vi "Wait n mSec.vi"(2 "Do Not Wait on Error?":bool=TRUE caption="Do NOT Wait on Error?\n(true)", 9 "Error in (no error)":errorcluster, 13 "Milliseconds to Wait (1)":u32=1 caption="mS") -> (10 "Error Out":errorcluster)   [LabVIEW 2015]
doc: "This VI allows you to drop in wait ms delays in your data-flow. Additionally it lets you specify if the wait should be skipped on errors (default) or if you want the wait to occur regardless of the error state!\nThe default wait value should be changed to suit your application."
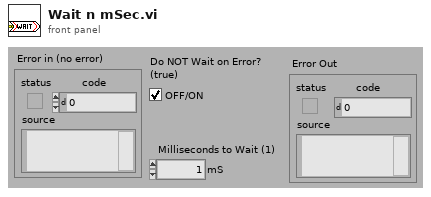
[diagram p1: front panel]
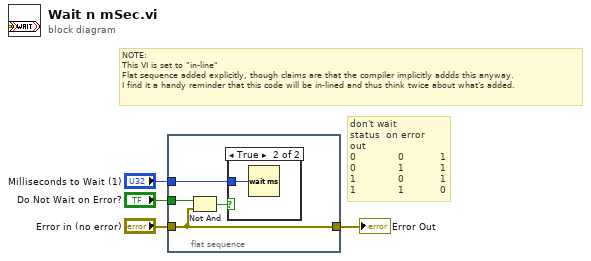
[diagram p0: block diagram]
diagram:
  # "don't wait  \nstatus  on error   out\n0              0            1\n0              1            1\n1              0            1\n1              1            0"
  # "NOTE:\nThis VI is set to \"in-line\"\nFlat sequence added explicitly, though claims are that the compiler implicitly addds this anyway.\nI find it a handy reminder that this code will be in-lined and thus think twice about what's added."
  n1 = flat-sequence {
    tunnel: "Milliseconds to Wait (1)" -> [w8]
    tunnel: [w6] -> w3
    tunnel: "Error in (no error)" -> [w6]
    tunnel: "Do Not Wait on Error?" -> [w7]
    frame #0 {
      n2 = Not And(1:w6, 2:w7) -> (0:w5:bool)
      n3 = case shown="True" w5 {
        tunnel: w8 -> [_ w9]
        frame False {
        }
        frame True {
          n4 = Wait (ms)(milliseconds to wait=w9) -> ()  [unwired: 1 out]
        }
      }
    }
  }
  "Error Out" <- w3
